vi "TelemetryDebug.vi"() -> ()   [LabVIEW 2020, in "VectoTools.lvlib" / "TelemetryDebug.lvclass"]
uses:
  TelemetryDebug/TelemetryDebug.lvclass
panel:
  in  "Start":bool
  in  "DiscoveryPort":u16=36986
  in  "Discovery Address":string="239.0.0.50"
  in  "Cluster":string="testCluster"
  in  "System":string="testSystem"
  in  "Tree":string(tree)
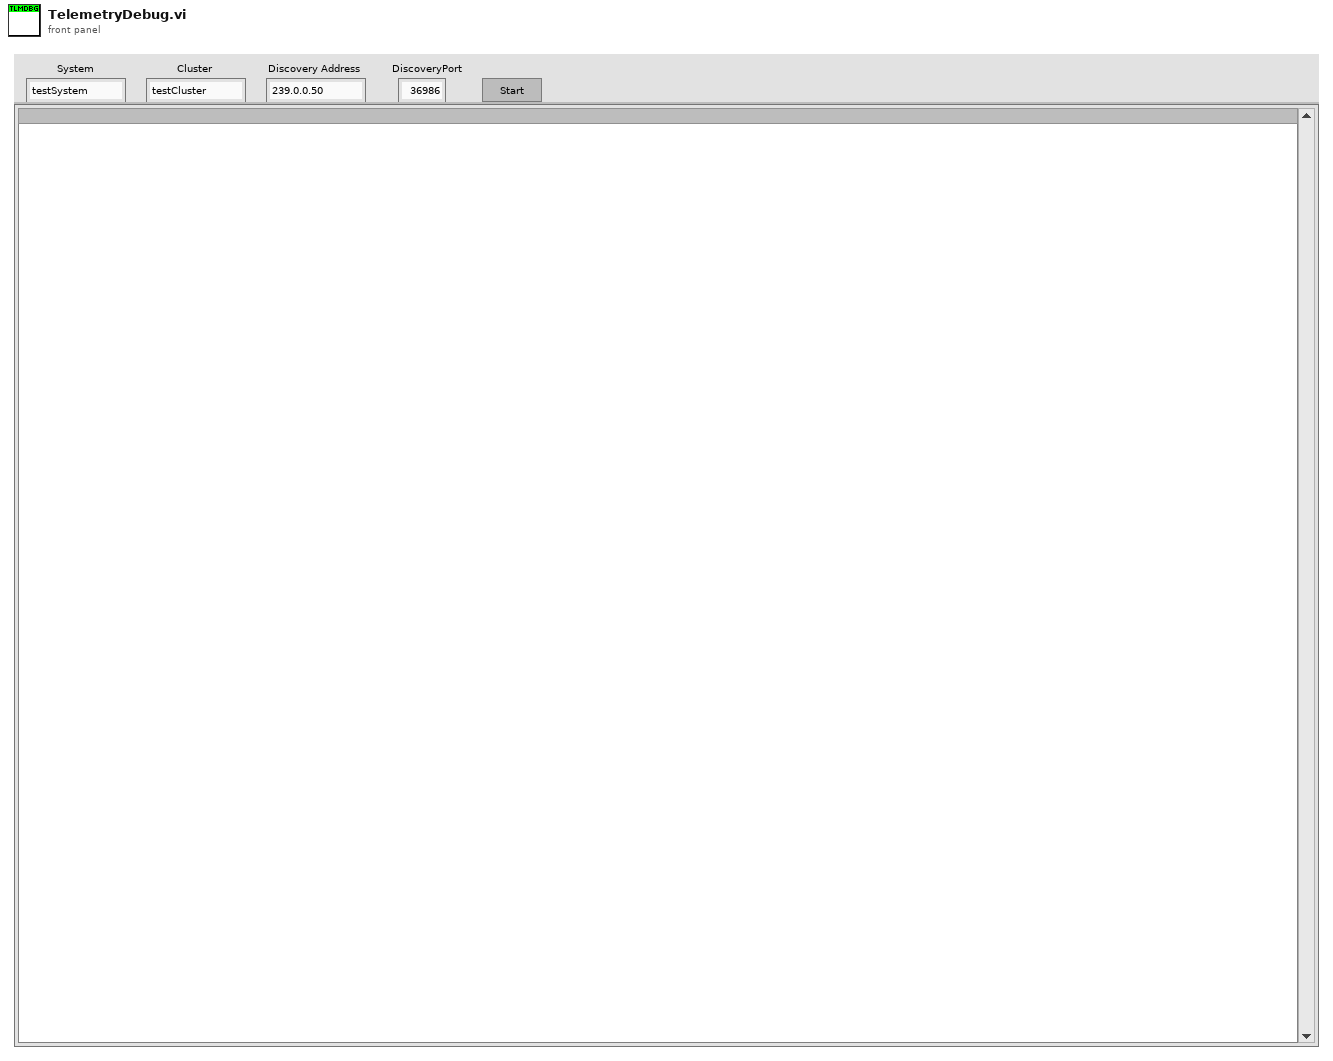
[diagram p1: front panel]
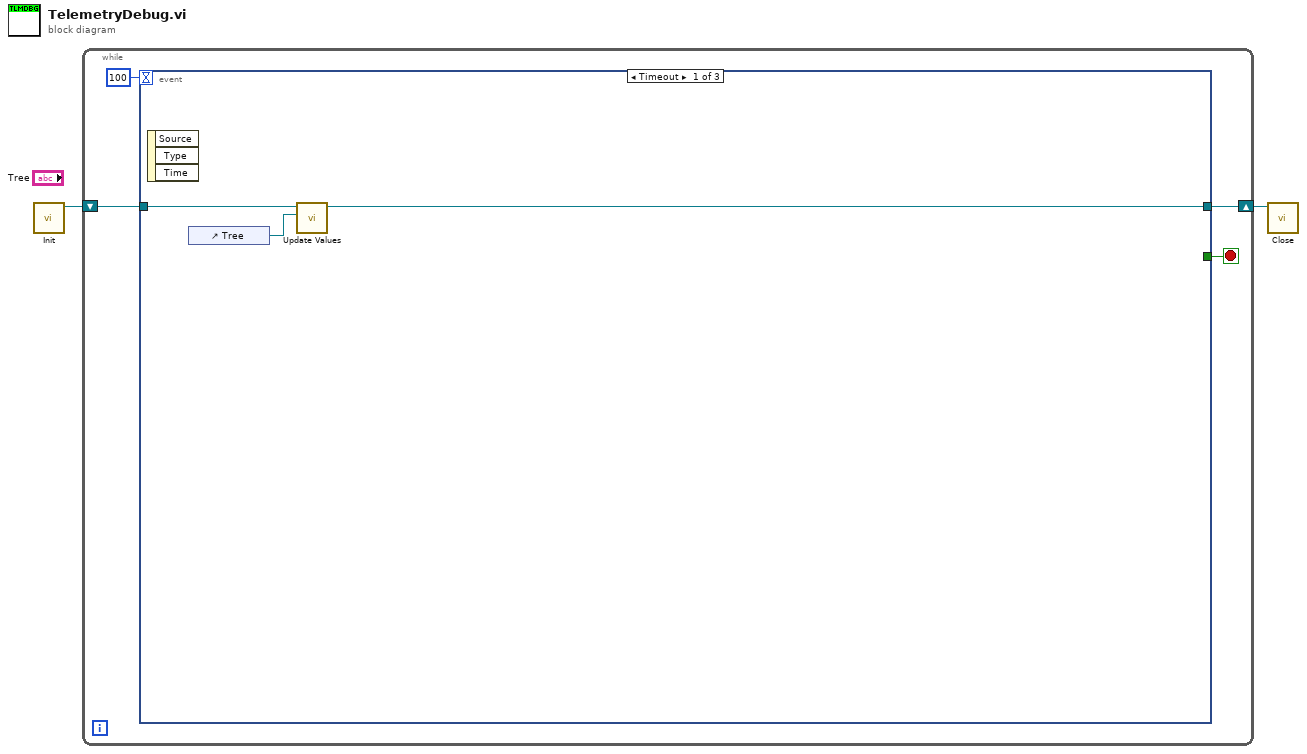
[diagram p0: block diagram]
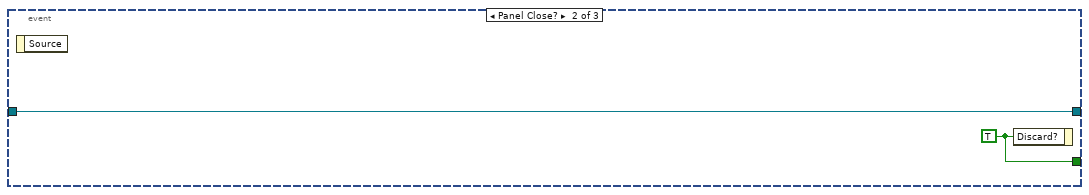
[diagram p2: hidden frame]
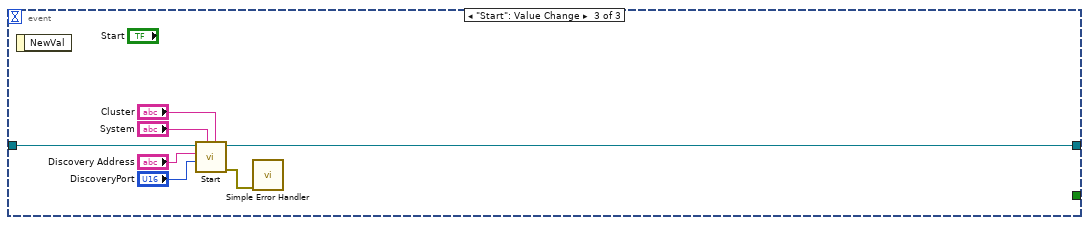
[diagram p3: hidden frame]
diagram:
  n1 = call "Init.vi"() -> ("TelemetryDebug out"=w2:refnum<class "TelemetryDebug.lvclass">)  [unwired: 10 in, 1 out]
  n2 = while {
    shift-right: [w4] -> w1
    shift-left: w2 -> [w5]
    stop <- w3 stop-if-true
    n3 = event shown="[0] Timeout" {
      selector: _ -> [_ _ _]
      dyn-events: _ -> [_ _ _]
      timeout: 100 -> [_ _ _]
      tunnel: w5 -> [w9 w11 w18]
      tunnel: [w8 w11 w17] -> w4
      tunnel: [_ w10 _] -> w3
      event Timeout {
        n4 = event-data() -> ()  [unwired: 1 in, 3 out]
        n5 = control-ref of="Tree"() -> (w7:refnum<vi>)
        n6 = call "Update Values.vi"("Tree"=w7, "TelemetryDebug in"=w9) -> ("TelemetryDebug out"=w8:refnum<class "TelemetryDebug.lvclass">)  [unwired: 8 in, 1 out]
      }
      event Panel Close? {
        w10 = TRUE ("Discard?")
        n7 = event-data() -> ()  [unwired: 1 in, 1 out]
        n8 = event-data("Discard?"=w10) -> ()  [unwired: 1 in, 1 out]
      }
      event "Start": Value Change {
        n9 = event-data() -> ()  [unwired: 1 in, 1 out]
        n10 = call "Start.vi"("Cluster"="Cluster", "System"="System", "DiscoveryPort"="DiscoveryPort", "Discovery Address"="Discovery Address", "TelemetryDebug in"=w18) -> ("error out"=w12:errorcluster, "TelemetryDebug out"=w17:refnum<class "TelemetryDebug.lvclass">)  [unwired: 5 in]
        n11 = call <vilib>:"Simple Error Handler.vi"("error in (no error)"=w12) -> ()  [unwired: 4 in, 5 out]
      }
    }
  }
  n12 = call "Close.vi"("TelemetryDebug in"=w1) -> ()  [unwired: 10 in, 1 out]
